vi "Write CLI Log Message.vi"(8 "error in (no error)":errorcluster {"code" format="Error %.0f"}, 10 "Message":string, 11 "DMC Folder Test Runner in":refnum<class "DMC Folder Test Runner.lvclass">) -> (0 "error out":errorcluster {"code" format="Error %.0f"}, 3 "DMC Folder Test Runner out":refnum<class "DMC Folder Test Runner.lvclass">)   [LabVIEW 2023, in "DMC Folder Test Runner.lvclass"]
uses:
  DMC Folder Test Runner.lvclass
  DMC Folder Test Runner.lvclass/DMC Folder Test Runner.ctl
  <vilib>/Wiresmith Technology/G CLI/CLI Class/CLI.lvclass
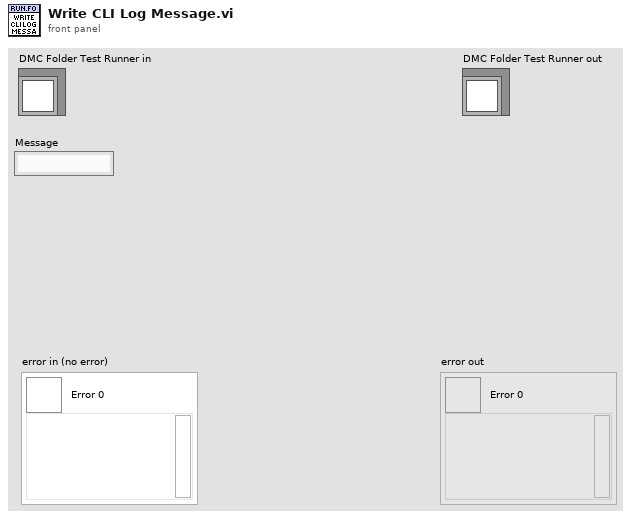
[diagram p1: front panel]
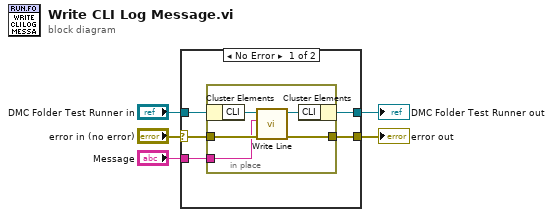
[diagram p0: block diagram]
diagram:
  n1 = case shown="No Error" "error in (no error)" {
    selector: "error in (no error)" -> [w10 w17]
    tunnel: [w6 w17] -> w3
    tunnel: [w9 w16] -> w2
    tunnel: "DMC Folder Test Runner in" -> [w8 w16]
    tunnel: "Message" -> [w7 _]
    frame No Error {
      n2 = in-place {
        in-place-border: w10 -> [w14]
        in-place-border: w7 -> [w13]
        in-place-border: [w11] -> w6
        n3 = in-place-cluster #1(w8) -> ("CLI"=w15:refnum<class "CLI.lvclass">)
        n4 = call <vilib>:"Write Line.vi"("error in (no error)"=w14, "Text to Write"=w13, "CLI in"=w15) -> ("error out"=w11:errorcluster, "CLI out"=w12:refnum<class "CLI.lvclass">)  [unwired: 7 in]
        n5 = in-place-cluster #1("CLI"=w12) -> (w9:refnum<class "DMC Folder Test Runner.lvclass">)
      }
    }
    frame Error {
    }
  }
  "error out" <- w3
  "DMC Folder Test Runner out" <- w2
